vi "Create.vi"(8 "error in (no error)":errorcluster, 11 "Messenger in":refnum<class "MGR.lvclass">) -> (0 "error out":errorcluster, 3 "Messenger out":refnum<class "MGR.lvclass">)   [LabVIEW 2011, in "Messenging.lvlib" / "MGR.lvclass"]
uses:
  MGR.lvclass
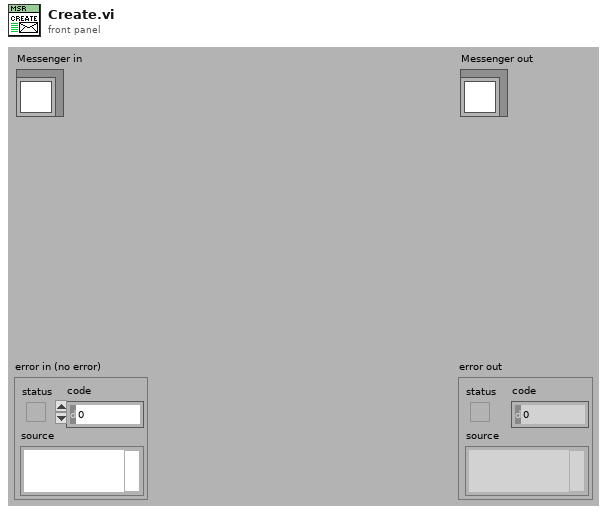
[diagram p1: front panel]
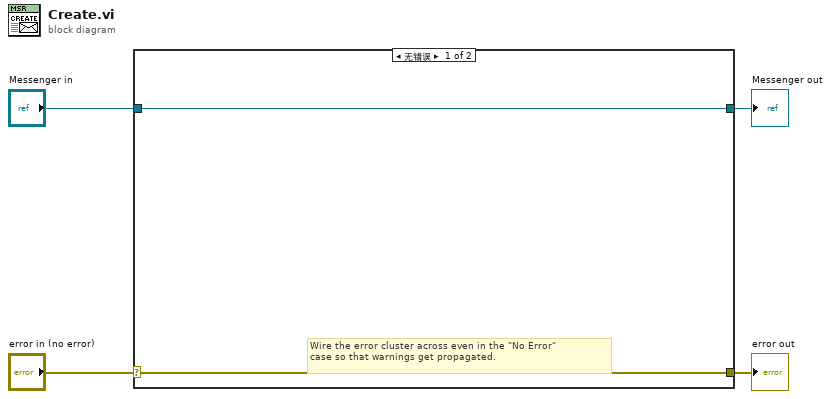
[diagram p0: block diagram]
diagram:
  n1 = case shown="无错误" "error in (no error)" {
    selector: "error in (no error)" -> [w5 w8]
    tunnel: [w5 w8] -> w3
    tunnel: [w6 w7] -> w1
    tunnel: "Messenger in" -> [w6 w7]
    frame No Error {
      # "Wire the error cluster across even in the \"No Error\"\ncase so that warnings get propagated."
    }
    frame Error {
    }
  }
  "error out" <- w3
  "Messenger out" <- w1
